vi "_070.vi"() -> ()   [LabVIEW 2024]
uses:
  <vilib>/express/express analysis/Spectral/XNode/ExpressSpectralMeasurementsBlockNode.xnode
  <vilib>/express/express analysis/Spectral/Block/exnSpectralBlock spectral measurements PSD poly.vi
  <vilib>/express/express analysis/Spectral/Block/exnSpectralBlock spectral measurements PSD DDT.vi
panel:
  out "Add":dynamicdata(graph)
  out "F2":dynamicdata(graph)
  out "F1":dynamicdata(graph)
  out "FF1":dynamicdata(graph)
  in  "stop":bool
  in  "F2":dbl(knob) scale=0.0..500.0
  in  "F1":dbl(knob) scale=0.0..500.0
  # "Time domain to frequency domain"
  # "( FFT - Fast Fourier Transform )"
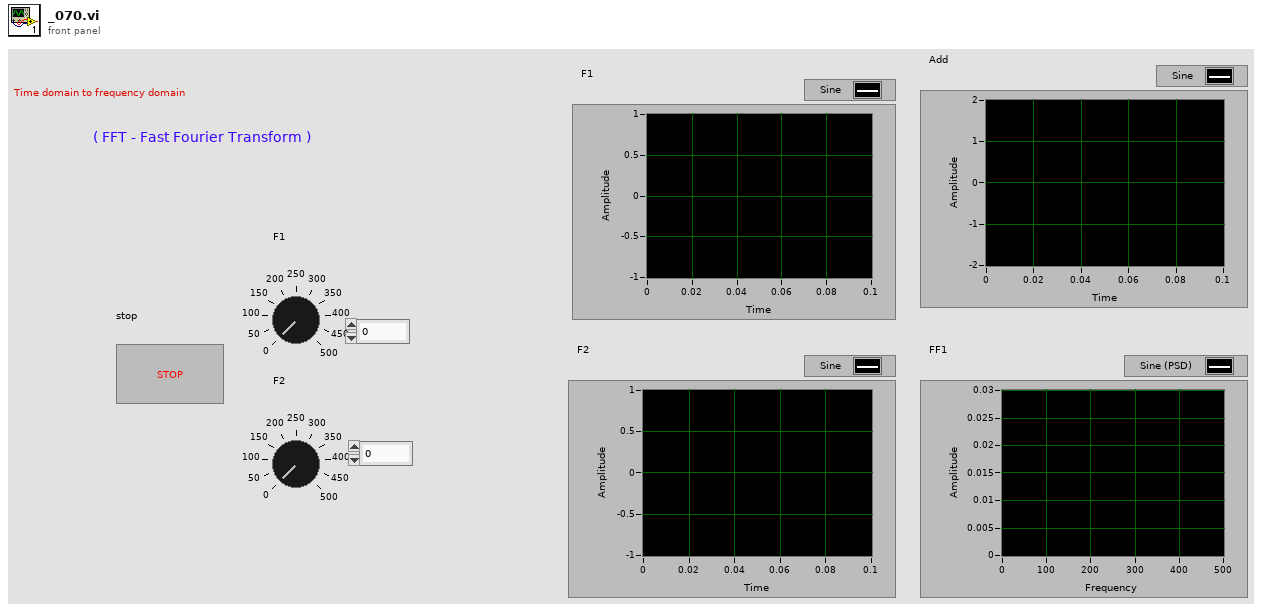
[diagram p1: front panel]
types:
  T1 = cluster{"averaging mode":u16, "weighting mode":u16, "number of averages":u32}
  T2 = cluster{"dB On (F)":bool, "unwrap phase (F)":bool, "convert to degree (F)":bool}
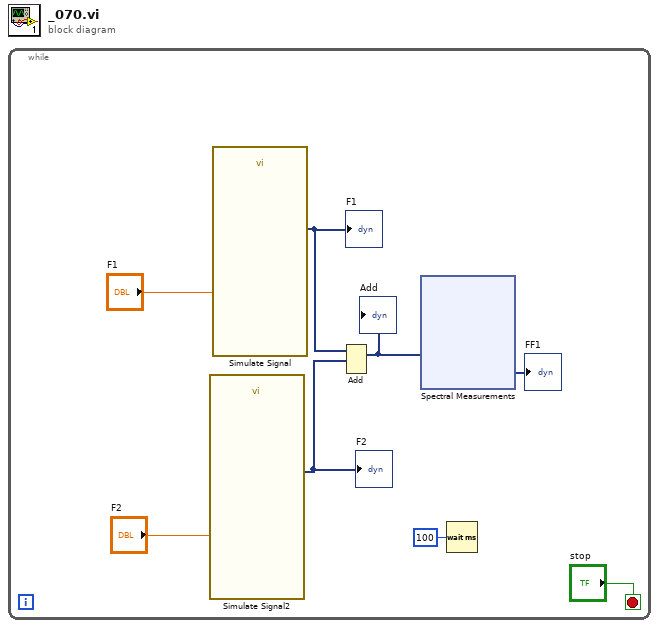
[diagram p0: block diagram]
diagram:
  n1 = while {
    stop <- "stop" stop-if-true
    n2 = call "Simulate Signal2"("Frequency"="F2") -> ("Sine"=w3:dynamicdata)  [unwired: 13 in, 1 out]
    "F2" <- w3
    n3 = call "Simulate Signal"("Frequency"="F1") -> ("Sine"=w4:dynamicdata)  [unwired: 13 in, 1 out]
    "F1" <- w4
    n4 = Add(1:w3, 2:w4) -> (0:w2:dynamicdata)  [unwired: 1 in, 1 out]
    "Add" <- w2
    n5 = xnode "Spectral Measurements"("Signals"=w2) -> ("PSD"=→"FF1":dynamicdata)  [unwired: 1 in, 1 out]
    n6 = Wait (ms)(milliseconds to wait=u32 100) -> ()  [unwired: 1 out]
  }
